vi "attempt-profileStaveCoreHeight.vi"() -> ()   [LabVIEW 2016]
uses:
  <vilib>/vision/driver/NI_Vision_Acquisition_Software.lvlib
  <vilib>/vision/NI_Vision_Development_Module.lvlib
  <vilib>/Utility/file.llb/Read Delimited Spreadsheet (DBL).vi
  <vilib>/Utility/file.llb/Write Delimited Spreadsheet (string).vi
  <vilib>/Utility/file.llb/Write Delimited Spreadsheet (DBL).vi
panel:
  out "True match index vector":i32[](array[numeric])=[1, 1, 1, 1, 1, 1, 1, 1, 1, 1, 1, 1, 1, 1, 1, 1, 1, 1, 1, 1, 1, 1, 1, 1, 1, 1, 1, 1, 1, 1, 1, 1, 1, 1, 1, 1, 1, 1, 1, 1, 1, 1, 1, 1, 1, 1, 1, 1, 1, 1, 1, 1, 1, 1, 1, 1, 1, 1, 1, 1, 1, 1, 1, 1, 1, 1, 1, 1, 1, 1, 1, 1, 1, 1, 1, 1, 1, 1, 1, 1, 1, 1, 1, 1, 1, 1, 1, 1, 1, 1, 1, 1, 1, 1, 1, 1, 1, 1, 1, 1, 1]
  in  "Save plots file path":path=path "E:/XYZstage+Camera_CollectedImages/12-14-2016"
  out "Z displacement [mm]":dbl[](array[numeric])=[-2.0, -1.9, -1.8, -1.7, -1.6, -1.5, -1.4, -1.2999999999999998, -1.2, -1.1, -1.0, -0.8999999999999999, -0.7999999999999998, -0.7, -0.5999999999999999, -0.5, -0.3999999999999999, -0.2999999999999998, -0.19999999999999996, -0.09999999999999987, 0.0, 0.10000000000000009, 0.20000000000000018, 0.30000000000000027, 0.40000000000000036, 0.5, 0.6000000000000001, 0.7000000000000002, 0.8000000000000003, 0.9000000000000004, 1.0, 1.1, 1.2000000000000002, 1.3000000000000003, 1.4000000000000004, 1.5, 1.6, 1.7000000000000002, 1.8000000000000003, 1.9000000000000004, 2.0, 2.1000000000000005, 2.2, 2.3, 2.4000000000000004, 2.5, 2.6000000000000005, 2.7, 2.8000000000000007, 2.9000000000000004, 3.0, 3.1000000000000005, 3.2, 3.3000000000000007, 3.4000000000000004, 3.5, 3.6000000000000005, 3.7, 3.8000000000000007, 3.9000000000000004, 4.0, 4.1000000000000005, 4.2, 4.300000000000001, 4.4, 4.5, 4.6000000000000005, 4.7, 4.800000000000001, 4.9, 5.0, 5.1000000000000005, 5.2, 5.300000000000001, 5.4, 5.5, 5.6000000000000005, 5.7, 5.800000000000001, 5.9, 6.0, 6.1, 6.200000000000001, 6.300000000000001, 6.4, 6.5, 6.6, 6.700000000000001, 6.800000000000001, 6.9, 7.0, 7.1, 7.200000000000001, 7.300000000000001, 7.4, 7.5, 7.600000000000001, 7.700000000000001, 7.800000000000001, 7.9, 8.0]
  out "Line Profile SD vs displacement":cluster{dbl[], sgl[]}(graph)={[-2.0, -1.9, -1.8, -1.7, -1.6, -1.5, -1.4, -1.2999999999999998, -1.2, -1.1, -1.0, -0.8999999999999999, -0.7999999999999998, -0.7, -0.5999999999999999, -0.5, -0.3999999999999999, -0.2999999999999998, -0.19999999999999996, -0.09999999999999987, 0.0, 0.10000000000000009, 0.20000000000000018, 0.30000000000000027, 0.40000000000000036, 0.5, 0.6000000000000001, 0.7000000000000002, 0.8000000000000003, 0.9000000000000004, 1.0, 1.1, 1.2000000000000002, 1.3000000000000003, 1.4000000000000004, 1.5, 1.6, 1.7000000000000002, 1.8000000000000003, 1.9000000000000004, 2.0, 2.1000000000000005, 2.2, 2.3, 2.4000000000000004, 2.5, 2.6000000000000005, 2.7, 2.8000000000000007, 2.9000000000000004, 3.0, 3.1000000000000005, 3.2, 3.3000000000000007, 3.4000000000000004, 3.5, 3.6000000000000005, 3.7, 3.8000000000000007, 3.9000000000000004, 4.0, 4.1000000000000005, 4.2, 4.300000000000001, 4.4, 4.5, 4.6000000000000005, 4.7, 4.800000000000001, 4.9, 5.0, 5.1000000000000005, 5.2, 5.300000000000001, 5.4, 5.5, 5.6000000000000005, 5.7, 5.800000000000001, 5.9, 6.0, 6.1, 6.200000000000001, 6.300000000000001, 6.4, 6.5, 6.6, 6.700000000000001, 6.800000000000001, 6.9, 7.0, 7.1, 7.200000000000001, 7.300000000000001, 7.4, 7.5, 7.600000000000001, 7.700000000000001, 7.800000000000001, 7.9, 8.0], [13.778814, 13.832154, 13.818352, 13.810552, 13.883811, 13.894283, 13.899467, 13.916209, 13.933476, 13.961703, 13.955698, 13.9895115, 13.971683, 14.028705, 14.043394, 14.072498, 14.079607, 14.094322, 14.10442, 14.146118, 14.114918, 14.148811, 14.173441, 14.218914, 14.194622, 14.272478, 14.306726, 14.26945, 14.336761, 14.362134, 14.373682, 14.395194, 14.455633, 14.497305, 14.4799185, 14.594659, 14.592479, 14.642527, 14.660905, 14.72331, 14.78993, 14.833229, 14.888031, 14.981282, 15.005414, 15.038977, 15.041095, 15.103504, 15.177525, 15.183865, 15.1743145, 15.172032, 15.142773, 15.190067, 15.161669, 15.174502, 15.0652895, 15.069694, 14.985318, 14.927153, 14.907353, 14.82682, 14.799372, 14.752344, 14.71759, 14.653623, 14.566762, 14.559869, 14.529179, 14.473595, 14.442641, 14.400999, 14.413042, 14.296873, 14.31068, 14.228256, 14.248779, 14.179554, 14.15682, 14.11064, 14.146657, 14.0807495, 14.068824, 14.026832, 14.009014, 14.026801, 14.005717, 13.982046, 13.993479, 13.971404, 13.941189, 13.940967, 13.946141, 13.935011, 13.897868, 13.873486, 13.894711, 13.855465, 13.869112, 13.84076, 13.822611]}
  in  "Line Profile Coordinates":i32[](array[numeric])=[0, 972, 2592, 972]
  out "Line Profile":cluster{"x0":sgl, "dx":sgl, "Pixels Line":sgl[]}(graph)={"x0"=0.0, "dx"=1.0, "Pixels Line"=[30.0, 30.0, 30.0, 29.0, 31.0, 30.0, 30.0, 30.0, 28.0, 30.0, 31.0, 31.0, 29.0, 31.0, 30.0, 31.0, 30.0, 29.0, 31.0, 32.0, 31.0, 31.0, 32.0, 32.0, 32.0, 32.0, 33.0, 33.0, 30.0, 35.0, 32.0, 32.0, 32.0, 33.0, 32.0, 35.0, 30.0, 34.0, 33.0, 34.0, 34.0, 34.0, 34.0, 34.0, 35.0, 35.0, 32.0, 34.0, 36.0, 36.0, 34.0, 36.0, 34.0, 35.0, 33.0, 38.0, 35.0, 34.0, 36.0, 35.0, 35.0, 37.0, 35.0, 37.0, 36.0, 33.0, 33.0, 37.0, 36.0, 37.0, 35.0, 37.0, 37.0, 36.0, 36.0, 37.0, 35.0, 37.0, 37.0, 33.0, 33.0, 35.0, 33.0, 33.0, 34.0, 34.0, 33.0, 34.0, 32.0, 34.0, 34.0, 34.0, 34.0, 35.0, 34.0, 35.0, 33.0, 34.0, 35.0, 34.0, 33.0, 34.0, 34.0, 33.0, 33.0, 32.0, 33.0, 34.0, 34.0, 31.0, 31.0, 31.0, 32.0, 31.0, 33.0, 32.0, 32.0, 31.0, 30.0, 31.0, 31.0, 33.0, 29.0, 32.0, 30.0, 31.0, 31.0, 32.0, 31.0, 30.0, 30.0, 32.0, 30.0, 31.0, 29.0, 31.0, 30.0, 29.0, 30.0, 30.0, 30.0, 31.0, 31.0, 31.0, 30.0, 32.0, 30.0, 31.0, 31.0, 30.0, 31.0, 31.0, 31.0, 33.0, 29.0, 31.0, 30.0, 31.0, 31.0, 32.0, 31.0, 32.0, 31.0, 30.0, 30.0, 31.0, 33.0, 31.0, 33.0, 33.0, 30.0, 33.0, 30.0, 34.0, 32.0, 33.0, 34.0, 34.0, 32.0, 34.0, 34.0, 34.0, 31.0, 36.0, 35.0, 34.0, 36.0, 31.0, 32.0, 33.0, 32.0, 34.0, 32.0, 33.0, 33.0, 33.0, 35.0, 34.0, 33.0, 33.0, 30.0, 36.0, 33.0, 31.0, 33.0, 32.0, 31.0, 33.0, 32.0, 33.0, 32.0, 33.0, 31.0, 31.0, 33.0, 31.0, 32.0, 32.0, 32.0, 32.0, 32.0, 31.0, 34.0, 33.0, 31.0, 33.0, 33.0, 35.0, 35.0, 34.0, 30.0, 34.0, 32.0, 33.0, 34.0, 34.0, 31.0, 32.0, 32.0, 32.0, 31.0, 32.0, 31.0, 31.0, 32.0, 32.0, 31.0, 33.0, 33.0, 31.0, 31.0, 34.0, 30.0, 35.0, 33.0, 33.0, 29.0, 33.0, 31.0, 32.0, 31.0, 33.0, 32.0, 32.0, 31.0, 32.0, 31.0, 33.0, 30.0, 31.0, 29.0, 30.0, 33.0, 31.0, 31.0, 29.0, 32.0, 32.0, 32.0, 29.0, 31.0, 33.0, 30.0, 32.0, 32.0, 31.0, 32.0, 31.0, 32.0, 31.0, 31.0, 32.0, 31.0, 31.0, 30.0, 32.0, 31.0, 32.0, 34.0, 30.0, 29.0, 33.0, 30.0, 30.0, 30.0, 33.0, 31.0, 31.0, 33.0, 32.0, 30.0, 31.0, 30.0, 32.0, 30.0, 32.0, 32.0, 33.0, 32.0, 34.0, 29.0, 33.0, 29.0, 32.0, 31.0, 32.0, 32.0, 32.0, 33.0, 33.0, 34.0, 32.0, 32.0, 34.0, 33.0, 34.0, 33.0, 34.0, 33.0, 36.0, 33.0, 33.0, 34.0, 34.0, 32.0, 35.0, 32.0, 33.0, 32.0, 32.0, 33.0, 31.0, 33.0, 33.0, 32.0, 36.0, 32.0, 32.0, 32.0, 34.0, 36.0, 32.0, 32.0, 34.0, 33.0, 35.0, 31.0, 32.0, 31.0, 34.0, 37.0, 32.0, 34.0, 35.0, 34.0, 32.0, 33.0, 34.0, 34.0, 34.0, 32.0, 37.0, 32.0, 35.0, 36.0, 35.0, 33.0, 32.0, 31.0, 35.0, 34.0, 34.0, 32.0, 34.0, 34.0, 34.0, 33.0, 33.0, 31.0, 33.0, 33.0, 33.0, 33.0, 34.0, 34.0, 34.0, 33.0, 35.0, 34.0, 34.0, 34.0, 36.0, 32.0, 36.0, 34.0, 35.0, 34.0, 34.0, 33.0, 34.0, 35.0, 37.0, 35.0, 34.0, 35.0, 36.0, 37.0, 36.0, 34.0, 32.0, 35.0, 33.0, 35.0, 35.0, 32.0, 35.0, 34.0, 33.0, 32.0, 33.0, 35.0, 34.0, 34.0, 32.0, 34.0, 33.0, 33.0, 32.0, 32.0, 32.0, 33.0, 33.0, 32.0, 34.0, 33.0, 34.0, 33.0, 34.0, 34.0, 35.0, 32.0, 35.0, 33.0, 33.0, 32.0, 32.0, 34.0, 34.0, 35.0, 34.0, 34.0, 34.0, 36.0, 35.0, 34.0, 35.0, 35.0, 36.0, 36.0, 37.0, 36.0, 35.0, 36.0, 35.0, 35.0, 34.0, 34.0, 35.0, 35.0, 35.0, 36.0, 38.0, 34.0, 34.0, 35.0, 36.0, 34.0, 35.0, 36.0, 35.0, 35.0, 36.0, 34.0, 36.0, 34.0, 36.0, 33.0, 32.0, 36.0, 36.0, 36.0, 35.0, 33.0, 36.0, 33.0, 32.0, 32.0, 35.0, 34.0, 35.0, 33.0, 35.0, 35.0, 34.0, 35.0, 35.0, 37.0, 34.0, 35.0, 35.0, 36.0, 35.0, 34.0, 35.0, 36.0, 35.0, 37.0, 37.0, 36.0, 39.0, 36.0, 37.0, 38.0, 37.0, 37.0, 35.0, 38.0, 40.0, 38.0, 40.0, 36.0, 39.0, 40.0, 37.0, 38.0, 41.0, 37.0, 41.0, 39.0, 41.0, 39.0, 41.0, 39.0, 40.0, 42.0, 40.0, 36.0, 40.0, 40.0, 40.0, 39.0, 40.0, 41.0, 39.0, 38.0, 39.0, 38.0, 39.0, 37.0, 35.0, 35.0, 36.0, 38.0, 36.0, 36.0, 35.0, 36.0, 34.0, 34.0, 35.0, 34.0, 36.0, 33.0, 34.0, 34.0, 32.0, 34.0, 34.0, 33.0, 35.0, 36.0, 35.0, 35.0, 35.0, 35.0, 33.0, 36.0, 33.0, 34.0, 34.0, 34.0, 35.0, 33.0, 35.0, 35.0, 37.0, 36.0, 35.0, 34.0, 33.0, 36.0, 35.0, 34.0, 35.0, 35.0, 34.0, 37.0, 34.0, 37.0, 34.0, 33.0, 35.0, 35.0, 35.0, 36.0, 34.0, 34.0, 35.0, 34.0, 36.0, 34.0, 35.0, 34.0, 35.0, 34.0, 34.0, 38.0, 35.0, 36.0, 37.0, 41.0, 38.0, 37.0, 36.0, 36.0, 39.0, 35.0, 38.0, 37.0, 35.0, 36.0, 36.0, 36.0, 35.0, 33.0, 35.0, 36.0, 32.0, 34.0, 34.0, 34.0, 33.0, 32.0, 30.0, 31.0, 32.0, 30.0, 33.0, 29.0, 31.0, 30.0, 28.0, 28.0, 29.0, 28.0, 28.0, 28.0, 27.0, 28.0, 26.0, 25.0, 24.0, 26.0, 28.0, 26.0, 29.0, 24.0, 25.0, 24.0, 23.0, 23.0, 22.0, 21.0, 20.0, 21.0, 20.0, 18.0, 20.0, 17.0, 19.0, 18.0, 17.0, 17.0, 17.0, 17.0, 15.0, 16.0, 16.0, 14.0, 14.0, 13.0, 12.0, 11.0, 13.0, 12.0, 11.0, 11.0, 11.0, 10.0, 10.0, 10.0, 9.0, 9.0, 9.0, 8.0, 8.0, 8.0, 9.0, 7.0, 7.0, 7.0, 7.0, 7.0, 7.0, 6.0, 6.0, 6.0, 7.0, 7.0, 6.0, 5.0, 6.0, 5.0, 5.0, 5.0, 5.0, 5.0, 5.0, 4.0, 4.0, 4.0, 4.0, 4.0, 4.0, 4.0, 3.0, 4.0, 4.0, 4.0, 3.0, 4.0, 3.0, 3.0, 4.0, 3.0, 3.0, 4.0, 3.0, 4.0, 3.0, 3.0, 3.0, 3.0, 3.0, 3.0, 3.0, 3.0, 3.0, 3.0, 3.0, 3.0, 2.0, 4.0, 3.0, 3.0, 3.0, 3.0, 3.0, 3.0, 3.0, 2.0, 3.0, 3.0, 3.0, 3.0, 2.0, 3.0, 2.0, 3.0, 3.0, 2.0, 3.0, 2.0, 2.0, 3.0, 3.0, 3.0, 3.0, 2.0, 3.0, 2.0, 4.0, 3.0, 3.0, 3.0, 3.0, 4.0, 4.0, 3.0, 3.0, 4.0, 4.0, 3.0, 3.0, 3.0, 4.0, 3.0, 3.0, 3.0, 4.0, 4.0, 3.0, 3.0, 4.0, 3.0, 4.0, 4.0, 3.0, 4.0, 4.0, 4.0, 3.0, 4.0, 4.0, 3.0, 3.0, 3.0, 4.0, 4.0, 4.0, 3.0, 3.0, 3.0, 4.0, 3.0, 3.0, 4.0, 3.0, 3.0, 3.0, 4.0, 3.0, 3.0, 3.0, 3.0, 3.0, 2.0, 3.0, 3.0, 2.0, 4.0, 4.0, 3.0, 3.0, 3.0, 3.0, 3.0, 3.0, 3.0, 3.0, 4.0, 3.0, 3.0, 3.0, 3.0, 3.0, 3.0, 3.0, 2.0, 3.0, 3.0, 3.0, 3.0, 3.0, 3.0, 4.0, 4.0, 3.0, 3.0, 2.0, 4.0, 4.0, 3.0, 3.0, 3.0, 3.0, 2.0, 3.0, 3.0, 3.0, 2.0, 4.0, 3.0, 4.0, 3.0, 3.0, 3.0, 3.0, 3.0, 3.0, 3.0, 3.0, 2.0, 3.0, 3.0, 3.0, 3.0, 4.0, 3.0, 3.0, 3.0, 3.0, 3.0, 4.0, 3.0, 3.0, 3.0, 3.0, 3.0, 4.0, 3.0, 3.0, 3.0, 3.0, 3.0, 3.0, 3.0, 4.0, 3.0, 5.0, 3.0, 5.0, 3.0, 3.0, 3.0, 4.0, 4.0, 4.0, 3.0, 4.0, 5.0, 4.0, 5.0, 6.0, 6.0, 6.0, 7.0, 8.0, 7.0, 7.0, 8.0, 10.0, 9.0, 11.0, 10.0, 13.0, 13.0, 13.0, 13.0, 14.0, 14.0, 16.0, 17.0, 19.0, 17.0, 18.0, 19.0, 19.0, 20.0, 22.0, 22.0, 21.0, 22.0, 21.0, 23.0, 25.0, 25.0, 26.0, 26.0, 29.0, 29.0, 30.0, 29.0, 28.0, 29.0, 32.0, 31.0, 31.0, 31.0, 35.0, 33.0, 35.0, 35.0, 33.0, 34.0, 35.0, 36.0, 35.0, 37.0, 37.0, 38.0, 40.0, 36.0, 40.0, 38.0, 40.0, 39.0, 37.0, 42.0, 41.0, 40.0, 41.0, 39.0, 41.0, 41.0, 42.0, 41.0, 38.0, 42.0, 42.0, 41.0, 40.0, 41.0, 44.0, 38.0, 41.0, 40.0, 43.0, 40.0, 44.0, 42.0, 41.0, 43.0, 43.0, 42.0, 41.0, 44.0, 44.0, 44.0, 45.0, 45.0, 43.0, 46.0, 44.0, 45.0, 42.0, 46.0, 44.0, 44.0, 43.0, 43.0, 46.0, 44.0, 45.0, 44.0, 44.0, 43.0, 44.0, 44.0, 45.0, 45.0, 44.0, 43.0, 43.0, 42.0, 42.0, 44.0, 43.0, 46.0, 43.0, 44.0, 42.0, 42.0, 44.0, 44.0, 43.0, 44.0, 45.0, 44.0, 47.0, 44.0, 46.0, 45.0, 43.0, 44.0, 44.0, 44.0, 43.0, 46.0, 42.0, 43.0, 46.0, 43.0, 47.0, 46.0, 48.0, 44.0, 48.0, 44.0, 43.0, 44.0, 43.0, 44.0, 46.0, 46.0, 45.0, 44.0, 50.0, 46.0, 45.0, 44.0, 45.0, 46.0, 45.0, 41.0, 46.0, 47.0, 47.0, 47.0, 48.0, 46.0, 47.0, 45.0, 44.0, 44.0, 46.0, 43.0, 48.0, 47.0, 45.0, 44.0, 43.0, 44.0, 44.0, 46.0, 46.0, 43.0, 43.0, 43.0, 44.0, 43.0, 44.0, 43.0, 45.0, 46.0, 46.0, 45.0, 45.0, 41.0, 44.0, 42.0, 45.0, 43.0, 47.0, 43.0, 48.0, 46.0, 46.0, 45.0, 46.0, 42.0, 47.0, 43.0, 45.0, 43.0, 45.0, 46.0, 46.0, 45.0, 46.0, 47.0, 47.0, 46.0, 49.0, 48.0, 48.0, 48.0, 50.0, 48.0, 49.0, 52.0, 51.0, 52.0, 52.0, 51.0, 53.0, 52.0, 50.0, 52.0, 50.0, 49.0, 50.0, 49.0, 49.0, 49.0, 54.0, 50.0, 47.0, 49.0, 46.0, 48.0, 48.0, 47.0, 50.0, 51.0, 50.0, 50.0, 49.0, 50.0, 50.0, 47.0, 47.0, 47.0, 44.0, 46.0, 46.0, 45.0, 45.0, 45.0, 47.0, 45.0, 45.0, 43.0, 41.0, 39.0, 37.0, 40.0, 37.0, 36.0, 35.0, 36.0, 37.0, 33.0, 35.0, 31.0, 33.0, 29.0, 27.0, 25.0, 27.0, 25.0, 24.0, 24.0, 24.0, 22.0, 22.0, 20.0, 19.0, 19.0, 18.0, 15.0, 15.0, 15.0, 15.0, 13.0, 12.0, 11.0, 12.0, 8.0, 8.0, 9.0, 8.0, 6.0, 7.0, 6.0, 6.0, 6.0, 5.0, 4.0, 5.0, 5.0, 3.0, 4.0, 5.0, 4.0, 4.0, 3.0, 5.0, 4.0, 3.0, 4.0, 3.0, 4.0, 3.0, 3.0, 3.0, 3.0, 4.0, 3.0, 3.0, 2.0, 4.0, 3.0, 3.0, 2.0, 2.0, 4.0, 3.0, 3.0, 3.0, 4.0, 3.0, 2.0, 3.0, 3.0, 3.0, 3.0, 3.0, 4.0, 3.0, 3.0, 3.0, 3.0, 3.0, 3.0, 3.0, 3.0, 3.0, 3.0, 3.0, 4.0, 3.0, 3.0, 3.0, 3.0, 3.0, 3.0, 3.0, 3.0, 3.0, 3.0, 2.0, 3.0, 3.0, 4.0, 3.0, 3.0, 4.0, 2.0, 3.0, 3.0, 3.0, 3.0, 3.0, 2.0, 3.0, 3.0, 4.0, 3.0, 3.0, 3.0, 3.0, 3.0, 3.0, 3.0, 3.0, 2.0, 3.0, 2.0, 4.0, 2.0, 3.0, 2.0, 3.0, 3.0, 3.0, 3.0, 3.0, 3.0, 3.0, 2.0, 3.0, 2.0, 3.0, 3.0, 3.0, 3.0, 3.0, 4.0, 3.0, 3.0, 3.0, 2.0, 3.0, 3.0, 3.0, 3.0, 3.0, 3.0, 3.0, 2.0, 3.0, 3.0, 3.0, 3.0, 3.0, 3.0, 3.0, 3.0, 3.0, 2.0, 3.0, 3.0, 2.0, 2.0, 3.0, 2.0, 3.0, 2.0, 3.0, 3.0, 2.0, 3.0, 2.0, 3.0, 3.0, 3.0, 3.0, 3.0, 3.0, 3.0, 3.0, 2.0, 3.0, 2.0, 2.0, 3.0, 3.0, 3.0, 3.0, 4.0, 4.0, 2.0, 3.0, 3.0, 3.0, 3.0, 2.0, 2.0, 2.0, 3.0, 2.0, 3.0, 2.0, 2.0, 2.0, 3.0, 3.0, 4.0, 3.0, 3.0, 3.0, 3.0, 3.0, 3.0, 2.0, 3.0, 3.0, 3.0, 3.0, 3.0, 3.0, 3.0, 3.0, 3.0, 3.0, 3.0, 2.0, 3.0, 3.0, 2.0, 3.0, 3.0, 4.0, 3.0, 3.0, 3.0, 3.0, 4.0, 3.0, 3.0, 4.0, 3.0, 3.0, 4.0, 4.0, 4.0, 5.0, 4.0, 5.0, 4.0, 5.0, 5.0, 5.0, 5.0, 6.0, 6.0, 6.0, 6.0, 6.0, 5.0, 7.0, 7.0, 7.0, 9.0, 7.0, 8.0, 9.0, 9.0, 9.0, 9.0, 9.0, 9.0, 9.0, 11.0, 11.0, 11.0, 11.0, 13.0, 13.0, 12.0, 15.0, 15.0, 14.0, 15.0, 16.0, 17.0, 18.0, 18.0, 21.0, 20.0, 20.0, 21.0, 21.0, 21.0, 23.0, 23.0, 23.0, 26.0, 26.0, 26.0, 28.0, 32.0, 30.0, 32.0, 33.0, 35.0, 36.0, 37.0, 35.0, 38.0, 38.0, 41.0, 41.0, 40.0, 43.0, 42.0, 44.0, 42.0, 42.0, 44.0, 42.0, 41.0, 41.0, 40.0, 38.0, 38.0, 40.0, 38.0, 38.0, 39.0, 37.0, 37.0, 38.0, 37.0, 37.0, 36.0, 36.0, 36.0, 36.0, 36.0, 37.0, 34.0, 36.0, 37.0, 38.0, 37.0, 36.0, 36.0, 38.0, 36.0, 36.0, 34.0, 36.0, 37.0, 36.0, 37.0, 36.0, 39.0, 37.0, 38.0, 38.0, 37.0, 40.0, 41.0, 40.0, 37.0, 38.0, 40.0, 40.0, 38.0, 37.0, 42.0, 40.0, 40.0, 39.0, 38.0, 40.0, 41.0, 40.0, 38.0, 40.0, 40.0, 40.0, 41.0, 41.0, 39.0, 39.0, 41.0, 42.0, 40.0, 42.0, 41.0, 40.0, 40.0, 40.0, 40.0, 40.0, 39.0, 41.0, 40.0, 41.0, 38.0, 38.0, 38.0, 40.0, 38.0, 38.0, 40.0, 36.0, 39.0, 39.0, 38.0, 37.0, 36.0, 38.0, 39.0, 39.0, 37.0, 39.0, 37.0, 40.0, 39.0, 38.0, 37.0, 39.0, 38.0, 37.0, 40.0, 40.0, 36.0, 38.0, 39.0, 39.0, 37.0, 39.0, 39.0, 40.0, 40.0, 41.0, 37.0, 40.0, 41.0, 39.0, 38.0, 40.0, 39.0, 39.0, 38.0, 41.0, 40.0, 38.0, 37.0, 38.0, 37.0, 39.0, 38.0, 38.0, 38.0, 37.0, 38.0, 36.0, 37.0, 38.0, 37.0, 36.0, 36.0, 39.0, 37.0, 35.0, 35.0, 37.0, 36.0, 34.0, 32.0, 34.0, 36.0, 34.0, 34.0, 36.0, 37.0, 35.0, 34.0, 36.0, 35.0, 37.0, 37.0, 36.0, 35.0, 34.0, 36.0, 35.0, 33.0, 35.0, 33.0, 35.0, 35.0, 36.0, 32.0, 36.0, 34.0, 34.0, 34.0, 34.0, 35.0, 33.0, 32.0, 33.0, 33.0, 32.0, 32.0, 31.0, 32.0, 32.0, 33.0, 31.0, 33.0, 32.0, 32.0, 32.0, 32.0, 34.0, 32.0, 34.0, 33.0, 33.0, 31.0, 33.0, 33.0, 32.0, 32.0, 31.0, 32.0, 33.0, 32.0, 30.0, 32.0, 31.0, 30.0, 32.0, 30.0, 30.0, 29.0, 29.0, 30.0, 28.0, 29.0, 32.0, 30.0, 29.0, 31.0, 30.0, 30.0, 30.0, 28.0, 29.0, 28.0, 28.0, 28.0, 30.0, 27.0, 27.0, 29.0, 27.0, 30.0, 28.0, 28.0, 30.0, 29.0, 29.0, 28.0, 27.0, 28.0, 28.0, 27.0, 25.0, 28.0, 29.0, 28.0, 27.0, 26.0, 25.0, 27.0, 27.0, 28.0, 26.0, 27.0, 27.0, 27.0, 27.0, 25.0, 28.0, 25.0, 25.0, 24.0, 25.0, 23.0, 26.0, 24.0, 25.0, 25.0, 25.0, 23.0, 26.0, 24.0, 25.0, 25.0, 25.0, 26.0, 25.0, 25.0, 26.0, 24.0, 24.0, 24.0, 24.0, 23.0, 24.0, 24.0, 23.0, 22.0, 24.0, 23.0, 21.0, 23.0, 22.0, 22.0, 21.0, 21.0, 21.0, 19.0, 19.0, 19.0, 19.0, 19.0, 21.0, 18.0, 18.0, 17.0, 19.0, 18.0, 18.0, 17.0, 17.0, 18.0, 17.0, 17.0, 18.0, 18.0, 19.0, 18.0, 17.0, 18.0, 17.0, 18.0, 17.0, 18.0, 18.0, 17.0, 17.0, 18.0, 19.0, 18.0, 18.0, 17.0, 18.0, 17.0, 16.0, 17.0, 17.0, 18.0, 17.0, 16.0, 16.0, 17.0, 17.0, 17.0, 17.0, 17.0, 17.0, 17.0, 16.0, 16.0, 16.0, 17.0, 17.0, 17.0, 17.0, 16.0, 16.0, 16.0, 17.0, 19.0, 17.0, 15.0, 15.0, 16.0, 17.0, 16.0, 17.0, 16.0, 15.0, 15.0, 16.0, 15.0, 15.0, 16.0, 17.0, 17.0, 15.0, 15.0, 16.0, 16.0, 17.0, 16.0, 16.0, 16.0, 17.0, 15.0, 17.0, 15.0, 16.0, 16.0, 15.0, 16.0, 15.0, 15.0, 16.0, 14.0, 15.0, 16.0, 17.0, 16.0, 16.0, 17.0, 16.0, 16.0, 18.0, 17.0, 15.0, 15.0, 15.0, 16.0, 16.0, 13.0, 16.0, 16.0, 16.0, 16.0, 16.0, 15.0, 16.0, 15.0, 16.0, 16.0, 16.0, 15.0, 15.0, 15.0, 17.0, 15.0, 16.0, 17.0, 16.0, 16.0, 17.0, 16.0, 17.0, 14.0, 15.0, 15.0, 16.0, 18.0, 14.0, 15.0, 15.0, 15.0, 17.0, 16.0, 16.0, 16.0, 14.0, 16.0, 15.0, 15.0, 14.0, 17.0, 15.0, 13.0, 15.0, 14.0, 14.0, 14.0, 15.0, 15.0, 15.0, 16.0, 14.0, 15.0, 15.0, 16.0, 15.0, 15.0, 15.0, 14.0, 15.0, 15.0, 14.0, 15.0, 14.0, 15.0, 15.0, 15.0, 16.0, 14.0, 15.0, 15.0, 15.0, 15.0, 15.0, 15.0, 15.0, 15.0, 15.0, 15.0, 14.0, 16.0, 15.0, 14.0, 14.0, 16.0, 14.0, 13.0, 15.0, 15.0, 15.0, 15.0, 15.0, 14.0, 14.0, 14.0, 15.0, 14.0, 15.0, 15.0, 15.0, 15.0, 15.0, 15.0, 15.0, 15.0, 15.0, 14.0, 15.0, 16.0, 16.0, 15.0, 15.0, 15.0, 17.0, 14.0, 16.0, 14.0, 15.0, 15.0, 13.0, 14.0, 16.0, 15.0, 15.0, 14.0, 16.0, 15.0, 15.0, 16.0, 16.0, 15.0, 15.0, 13.0, 16.0, 15.0, 14.0, 14.0, 14.0, 14.0, 15.0, 15.0, 13.0, 15.0, 15.0, 16.0, 14.0, 13.0, 14.0, 15.0, 14.0, 15.0, 15.0, 14.0, 15.0, 13.0, 16.0, 13.0, 15.0, 13.0, 14.0, 14.0, 13.0, 15.0, 15.0, 14.0, 15.0, 15.0, 15.0, 14.0, 15.0, 14.0, 14.0, 14.0, 14.0, 15.0, 14.0, 15.0, 14.0, 14.0, 13.0, 15.0, 14.0, 14.0, 15.0, 13.0, 13.0, 14.0, 14.0, 14.0, 15.0, 13.0, 14.0, 12.0, 13.0, 12.0, 13.0, 13.0, 13.0, 13.0, 11.0, 13.0, 13.0, 13.0, 13.0, 13.0, 12.0, 12.0, 12.0, 14.0, 14.0, 15.0, 13.0, 13.0, 13.0, 13.0, 13.0, 13.0, 14.0, 14.0, 14.0, 13.0, 13.0, 12.0, 13.0, 12.0, 13.0, 14.0, 13.0, 13.0, 13.0, 14.0, 14.0, 12.0, 13.0, 13.0, 14.0, 12.0, 13.0, 14.0, 14.0, 12.0, 15.0, 13.0, 13.0, 12.0, 14.0, 13.0, 13.0, 13.0, 14.0, 13.0, 14.0, 13.0, 14.0, 14.0, 15.0, 13.0, 14.0, 14.0, 14.0, 14.0, 13.0, 13.0, 14.0, 13.0, 13.0, 12.0, 13.0, 14.0, 13.0, 13.0, 13.0, 12.0, 12.0, 13.0, 13.0, 13.0, 13.0, 12.0, 15.0, 11.0, 13.0, 12.0, 12.0, 11.0, 14.0, 12.0, 14.0, 12.0, 14.0, 13.0, 12.0, 12.0, 12.0, 13.0, 12.0, 12.0, 13.0, 12.0, 12.0, 13.0, 13.0, 12.0, 13.0, 13.0, 13.0, 13.0, 13.0, 13.0, 13.0, 13.0, 12.0, 10.0, 14.0, 12.0, 11.0, 11.0, 12.0, 12.0, 13.0, 13.0, 12.0, 12.0, 13.0, 12.0, 12.0, 12.0, 12.0, 11.0, 13.0, 12.0, 12.0, 14.0, 12.0, 13.0, 13.0, 11.0, 12.0, 12.0, 12.0, 12.0, 12.0, 13.0, 12.0, 11.0, 14.0, 13.0, 13.0, 13.0, 12.0, 12.0, 12.0, 12.0, 13.0, 12.0, 13.0, 12.0, 13.0, 13.0, 12.0, 12.0, 13.0, 11.0, 12.0, 13.0, 14.0, 14.0, 11.0, 13.0, 13.0, 11.0, 11.0, 12.0, 13.0, 13.0, 13.0, 13.0, 12.0, 12.0, 12.0, 11.0, 12.0, 12.0, 12.0, 13.0, 14.0, 14.0, 14.0, 13.0, 13.0, 12.0, 13.0, 12.0, 12.0, 13.0, 13.0, 12.0, 14.0, 13.0, 12.0, 12.0, 13.0, 12.0, 14.0, 14.0, 13.0, 13.0, 13.0, 13.0, 13.0, 12.0, 13.0, 13.0, 13.0, 14.0, 13.0, 14.0, 15.0, 12.0, 13.0, 13.0, 14.0, 13.0, 13.0, 12.0, 12.0, 14.0, 12.0, 13.0, 14.0, 14.0, 14.0, 13.0, 13.0, 13.0, 14.0, 13.0, 14.0, 14.0, 15.0, 12.0, 14.0, 14.0, 13.0, 13.0, 13.0, 13.0, 15.0, 15.0, 13.0, 13.0, 15.0, 15.0, 14.0, 14.0, 13.0, 15.0, 15.0, 13.0, 13.0, 15.0, 13.0, 13.0, 15.0, 15.0, 13.0, 14.0, 13.0, 12.0, 14.0, 12.0, 14.0, 14.0, 14.0, 14.0, 13.0, 13.0, 15.0, 13.0, 13.0, 14.0, 15.0, 14.0, 13.0, 13.0, 14.0, 14.0, 14.0, 15.0, 14.0, 13.0, 15.0, 15.0, 14.0, 13.0, 15.0, 15.0, 15.0, 15.0, 14.0, 13.0, 15.0, 14.0, 14.0, 14.0, 14.0, 13.0, 14.0, 15.0, 15.0, 14.0, 13.0, 15.0, 15.0, 14.0, 14.0, 15.0, 15.0, 13.0, 14.0, 14.0, 14.0, 15.0, 15.0, 13.0, 15.0, 13.0, 14.0, 13.0, 14.0, 14.0, 14.0, 15.0, 14.0, 15.0, 15.0, 14.0, 15.0, 14.0, 13.0, 13.0, 14.0, 14.0, 13.0, 12.0, 14.0, 12.0, 14.0, 13.0, 14.0, 14.0, 14.0, 15.0, 14.0, 14.0, 14.0, 15.0, 15.0, 14.0, 14.0, 14.0, 15.0, 14.0, 14.0, 14.0, 15.0, 14.0, 14.0, 15.0, 14.0, 15.0, 15.0, 13.0, 16.0, 14.0, 15.0]}
  out "Coord. Index":i32
  in  "Process list?":bool
  in  "List of Interesting Locations":path=path "E:/XYZstage+Camera_CollectedImages/12-14-2016/nominalPOS_HighVoltageContacts.csv"
  in  "File delimiter":string=","
  out "Set of Coordinates to Process":dbl[][](array[numeric])=[[-709.0, -32.0, -2.0], [-611.0, -32.0, -2.0], [-513.0, -32.0, -2.0], [-415.0, -32.0, -2.0], [-317.0, -32.0, -2.0], [-219.0, -32.0, -2.0], [-121.0, -32.0, -2.0], [-23.0, -32.0, -2.0], [75.0, -32.0, -2.0], [173.0, -32.0, -2.0], [271.0, -32.0, -2.0], [369.0, -32.0, -2.0], [467.0, -32.0, -2.0], [467.0, -132.0, -2.0], [369.0, -132.0, -2.0], [271.0, -132.0, -2.0], [173.0, -132.0, -2.0], [75.0, -132.0, -2.0], [-23.0, -132.0, -2.0], [-121.0, -132.0, -2.0], [-219.0, -132.0, -2.0], [-317.0, -132.0, -2.0], [-415.0, -132.0, -2.0], [-513.0, -132.0, -2.0], [-611.0, -132.0, -2.0], [-709.0, -132.0, -2.0]]
  out "True match index vs displacement":cluster{dbl[], i32[]}(graph)={[-2.0, -1.9, -1.8, -1.7, -1.6, -1.5, -1.4, -1.2999999999999998, -1.2, -1.1, -1.0, -0.8999999999999999, -0.7999999999999998, -0.7, -0.5999999999999999, -0.5, -0.3999999999999999, -0.2999999999999998, -0.19999999999999996, -0.09999999999999987, 0.0, 0.10000000000000009, 0.20000000000000018, 0.30000000000000027, 0.40000000000000036, 0.5, 0.6000000000000001, 0.7000000000000002, 0.8000000000000003, 0.9000000000000004, 1.0, 1.1, 1.2000000000000002, 1.3000000000000003, 1.4000000000000004, 1.5, 1.6, 1.7000000000000002, 1.8000000000000003, 1.9000000000000004, 2.0, 2.1000000000000005, 2.2, 2.3, 2.4000000000000004, 2.5, 2.6000000000000005, 2.7, 2.8000000000000007, 2.9000000000000004, 3.0, 3.1000000000000005, 3.2, 3.3000000000000007, 3.4000000000000004, 3.5, 3.6000000000000005, 3.7, 3.8000000000000007, 3.9000000000000004, 4.0, 4.1000000000000005, 4.2, 4.300000000000001, 4.4, 4.5, 4.6000000000000005, 4.7, 4.800000000000001, 4.9, 5.0, 5.1000000000000005, 5.2, 5.300000000000001, 5.4, 5.5, 5.6000000000000005, 5.7, 5.800000000000001, 5.9, 6.0, 6.1, 6.200000000000001, 6.300000000000001, 6.4, 6.5, 6.6, 6.700000000000001, 6.800000000000001, 6.9, 7.0, 7.1, 7.200000000000001, 7.300000000000001, 7.4, 7.5, 7.600000000000001, 7.700000000000001, 7.800000000000001, 7.9, 8.0], [1, 1, 1, 1, 1, 1, 1, 1, 1, 1, 1, 1, 1, 1, 1, 1, 1, 1, 1, 1, 1, 1, 1, 1, 1, 1, 1, 1, 1, 1, 1, 1, 1, 1, 1, 1, 1, 1, 1, 1, 1, 1, 1, 1, 1, 1, 1, 1, 1, 1, 1, 1, 1, 1, 1, 1, 1, 1, 1, 1, 1, 1, 1, 1, 1, 1, 1, 1, 1, 1, 1, 1, 1, 1, 1, 1, 1, 1, 1, 1, 1, 1, 1, 1, 1, 1, 1, 1, 1, 1, 1, 1, 1, 1, 1, 1, 1, 1, 1, 1, 1]}
  in  "True position y":sgl=919.0
  in  "True position x":sgl=1107.0
  out "SD Intensity":cluster{dbl[], sgl[]}(graph)={[-2.0, -1.9, -1.8, -1.7, -1.6, -1.5, -1.4, -1.2999999999999998, -1.2, -1.1, -1.0, -0.8999999999999999, -0.7999999999999998, -0.7, -0.5999999999999999, -0.5, -0.3999999999999999, -0.2999999999999998, -0.19999999999999996, -0.09999999999999987, 0.0, 0.10000000000000009, 0.20000000000000018, 0.30000000000000027, 0.40000000000000036, 0.5, 0.6000000000000001, 0.7000000000000002, 0.8000000000000003, 0.9000000000000004, 1.0, 1.1, 1.2000000000000002, 1.3000000000000003, 1.4000000000000004, 1.5, 1.6, 1.7000000000000002, 1.8000000000000003, 1.9000000000000004, 2.0, 2.1000000000000005, 2.2, 2.3, 2.4000000000000004, 2.5, 2.6000000000000005, 2.7, 2.8000000000000007, 2.9000000000000004, 3.0, 3.1000000000000005, 3.2, 3.3000000000000007, 3.4000000000000004, 3.5, 3.6000000000000005, 3.7, 3.8000000000000007, 3.9000000000000004, 4.0, 4.1000000000000005, 4.2, 4.300000000000001, 4.4, 4.5, 4.6000000000000005, 4.7, 4.800000000000001, 4.9, 5.0, 5.1000000000000005, 5.2, 5.300000000000001, 5.4, 5.5, 5.6000000000000005, 5.7, 5.800000000000001, 5.9, 6.0, 6.1, 6.200000000000001, 6.300000000000001, 6.4, 6.5, 6.6, 6.700000000000001, 6.800000000000001, 6.9, 7.0, 7.1, 7.200000000000001, 7.300000000000001, 7.4, 7.5, 7.600000000000001, 7.700000000000001, 7.800000000000001, 7.9, 8.0], [10.641642, 10.651783, 10.666476, 10.678297, 10.692045, 10.704219, 10.71487, 10.729536, 10.741039, 10.750571, 10.763839, 10.775967, 10.788582, 10.799376, 10.81211, 10.824463, 10.83405, 10.845817, 10.859667, 10.870168, 10.882172, 10.89403, 10.906297, 10.919101, 10.931665, 10.943659, 10.956027, 10.969385, 10.981974, 10.995705, 11.010284, 11.024967, 11.0413475, 11.057471, 11.074867, 11.091722, 11.112195, 11.129671, 11.15188, 11.172808, 11.193802, 11.216489, 11.236443, 11.253368, 11.273286, 11.291981, 11.304524, 11.317779, 11.327574, 11.333745, 11.336129, 11.336787, 11.332882, 11.329793, 11.322591, 11.313084, 11.304098, 11.292609, 11.283385, 11.271473, 11.260806, 11.251673, 11.241544, 11.231288, 11.225223, 11.217907, 11.210427, 11.205402, 11.200951, 11.193987, 11.189045, 11.183764, 11.177903, 11.175188, 11.171228, 11.166864, 11.165156, 11.162128, 11.160154, 11.158059, 11.1588125, 11.157321, 11.157779, 11.158607, 11.159854, 11.16267, 11.164532, 11.167459, 11.167222, 11.171898, 11.173964, 11.176909, 11.17766, 11.180899, 11.182198, 11.1821165, 11.183969, 11.183027, 11.185584, 11.186689, 11.18563]}
  out "Mean intensity":cluster{dbl[], sgl[]}(graph)={[-2.0, -1.9, -1.8, -1.7, -1.6, -1.5, -1.4, -1.2999999999999998, -1.2, -1.1, -1.0, -0.8999999999999999, -0.7999999999999998, -0.7, -0.5999999999999999, -0.5, -0.3999999999999999, -0.2999999999999998, -0.19999999999999996, -0.09999999999999987, 0.0, 0.10000000000000009, 0.20000000000000018, 0.30000000000000027, 0.40000000000000036, 0.5, 0.6000000000000001, 0.7000000000000002, 0.8000000000000003, 0.9000000000000004, 1.0, 1.1, 1.2000000000000002, 1.3000000000000003, 1.4000000000000004, 1.5, 1.6, 1.7000000000000002, 1.8000000000000003, 1.9000000000000004, 2.0, 2.1000000000000005, 2.2, 2.3, 2.4000000000000004, 2.5, 2.6000000000000005, 2.7, 2.8000000000000007, 2.9000000000000004, 3.0, 3.1000000000000005, 3.2, 3.3000000000000007, 3.4000000000000004, 3.5, 3.6000000000000005, 3.7, 3.8000000000000007, 3.9000000000000004, 4.0, 4.1000000000000005, 4.2, 4.300000000000001, 4.4, 4.5, 4.6000000000000005, 4.7, 4.800000000000001, 4.9, 5.0, 5.1000000000000005, 5.2, 5.300000000000001, 5.4, 5.5, 5.6000000000000005, 5.7, 5.800000000000001, 5.9, 6.0, 6.1, 6.200000000000001, 6.300000000000001, 6.4, 6.5, 6.6, 6.700000000000001, 6.800000000000001, 6.9, 7.0, 7.1, 7.200000000000001, 7.300000000000001, 7.4, 7.5, 7.600000000000001, 7.700000000000001, 7.800000000000001, 7.9, 8.0], [20.910046, 20.920034, 20.933973, 20.943743, 20.955025, 20.964808, 20.9742, 20.98869, 20.994587, 21.002455, 21.015623, 21.023836, 21.03432, 21.04218, 21.053076, 21.061861, 21.071775, 21.081497, 21.091366, 21.098965, 21.109715, 21.117125, 21.126795, 21.136934, 21.146261, 21.154997, 21.164537, 21.172298, 21.18154, 21.189453, 21.19927, 21.211632, 21.220724, 21.229343, 21.23793, 21.247366, 21.258081, 21.265568, 21.273588, 21.283756, 21.294106, 21.302652, 21.31348, 21.320198, 21.327011, 21.338882, 21.345778, 21.358772, 21.366032, 21.376537, 21.384182, 21.392761, 21.40514, 21.417728, 21.425573, 21.433475, 21.441751, 21.451128, 21.459505, 21.468637, 21.47673, 21.483612, 21.492018, 21.49752, 21.503105, 21.509392, 21.514872, 21.523632, 21.529394, 21.531126, 21.542875, 21.543736, 21.54888, 21.55595, 21.561668, 21.567684, 21.575727, 21.58373, 21.591654, 21.598585, 21.611357, 21.617191, 21.631332, 21.643969, 21.65866, 21.672548, 21.685982, 21.70223, 21.714117, 21.73156, 21.747263, 21.763897, 21.775932, 21.792603, 21.805487, 21.818777, 21.831142, 21.844866, 21.861055, 21.877483, 21.887157]}
  out "Match score vs displacement":cluster{dbl[], sgl[]}(graph)={[-2.0, -1.9, -1.8, -1.7, -1.6, -1.5, -1.4, -1.2999999999999998, -1.2, -1.1, -1.0, -0.8999999999999999, -0.7999999999999998, -0.7, -0.5999999999999999, -0.5, -0.3999999999999999, -0.2999999999999998, -0.19999999999999996, -0.09999999999999987, 0.0, 0.10000000000000009, 0.20000000000000018, 0.30000000000000027, 0.40000000000000036, 0.5, 0.6000000000000001, 0.7000000000000002, 0.8000000000000003, 0.9000000000000004, 1.0, 1.1, 1.2000000000000002, 1.3000000000000003, 1.4000000000000004, 1.5, 1.6, 1.7000000000000002, 1.8000000000000003, 1.9000000000000004, 2.0, 2.1000000000000005, 2.2, 2.3, 2.4000000000000004, 2.5, 2.6000000000000005, 2.7, 2.8000000000000007, 2.9000000000000004, 3.0, 3.1000000000000005, 3.2, 3.3000000000000007, 3.4000000000000004, 3.5, 3.6000000000000005, 3.7, 3.8000000000000007, 3.9000000000000004, 4.0, 4.1000000000000005, 4.2, 4.300000000000001, 4.4, 4.5, 4.6000000000000005, 4.7, 4.800000000000001, 4.9, 5.0, 5.1000000000000005, 5.2, 5.300000000000001, 5.4, 5.5, 5.6000000000000005, 5.7, 5.800000000000001, 5.9, 6.0, 6.1, 6.200000000000001, 6.300000000000001, 6.4, 6.5, 6.6, 6.700000000000001, 6.800000000000001, 6.9, 7.0, 7.1, 7.200000000000001, 7.300000000000001, 7.4, 7.5, 7.600000000000001, 7.700000000000001, 7.800000000000001, 7.9, 8.0], [879.0314, 880.5322, 881.50525, 883.59375, 885.04114, 886.6321, 887.99164, 889.89014, 891.54895, 892.7096, 894.01355, 895.76086, 896.38574, 897.8513, 899.14215, 900.46564, 901.9159, 903.5967, 905.61066, 907.6271, 909.8519, 911.7539, 914.30066, 916.9432, 919.2109, 922.02893, 925.1449, 927.1994, 930.3543, 933.7616, 937.412, 941.27527, 945.56866, 949.7169, 954.40594, 958.87146, 964.12915, 966.3607, 971.17303, 975.7742, 979.7761, 983.59674, 986.48694, 988.4218, 989.78876, 991.7045, 990.82227, 992.4532, 993.7908, 994.56085, 994.9838, 995.4237, 995.7052, 996.1429, 996.40594, 995.1158, 994.9518, 994.49426, 993.5686, 991.30493, 988.9285, 985.62024, 979.23346, 976.25146, 972.1395, 967.325, 962.50824, 957.11816, 951.9495, 947.2621, 943.3269, 939.42737, 936.4822, 934.05096, 931.73193, 929.0479, 926.9251, 923.81866, 921.44275, 919.72864, 917.4266, 914.7757, 913.0611, 911.3056, 910.391, 910.2793, 909.92053, 909.1891, 908.61414, 907.92114, 906.2847, 905.24835, 904.1167, 902.81866, 901.4715, 900.2599, 898.7702, 897.3308, 896.09454, 894.80115, 893.3429]}
  in  "Match position variation tolerance":sgl=0.25
  out "Z step":dbl=10.0
  out "Image":T1(plugin-control)
  in  "End Z [mm]":dbl=8.0
  in  "Stepsize [mm]":dbl=0.1
  out "Matches (pixel)":T2(array[cluster])=[{"Position"={"x"=1127.198, "y"=915.98065}, "Angle"=0.0, "Scale"=1.0, "Score"=893.3429, "Bounding Box"=[{"x"=974.198, "y"=763.98065}, {"x"=1280.198, "y"=763.98065}, {"x"=1280.198, "y"=1067.9807}, {"x"=974.198, "y"=1067.9807}, {"x"=974.198, "y"=763.98065}]}, {"Position"={"x"=1514.1495, "y"=359.13376}, "Angle"=0.0, "Scale"=1.0, "Score"=588.01715, "Bounding Box"=[{"x"=1361.1495, "y"=207.13376}, {"x"=1667.1495, "y"=207.13376}, {"x"=1667.1495, "y"=511.13376}, {"x"=1361.1495, "y"=511.13376}, {"x"=1361.1495, "y"=207.13376}]}, {"Position"={"x"=530.31506, "y"=1381.0135}, "Angle"=0.0, "Scale"=1.0, "Score"=572.6888, "Bounding Box"=[{"x"=377.31506, "y"=1229.0135}, {"x"=683.31506, "y"=1229.0135}, {"x"=683.31506, "y"=1533.0135}, {"x"=377.31506, "y"=1533.0135}, {"x"=377.31506, "y"=1229.0135}]}, {"Position"={"x"=1194.1893, "y"=1528.8197}, "Angle"=0.0, "Scale"=1.0, "Score"=556.0711, "Bounding Box"=[{"x"=1041.1893, "y"=1376.8197}, {"x"=1347.1893, "y"=1376.8197}, {"x"=1347.1893, "y"=1680.8197}, {"x"=1041.1893, "y"=1680.8197}, {"x"=1041.1893, "y"=1376.8197}]}, {"Position"={"x"=129.51509, "y"=1364.8577}, "Angle"=0.0, "Scale"=1.0, "Score"=534.0569, "Bounding Box"=[{"x"=-23.48491, "y"=1212.8577}, {"x"=282.51508, "y"=1212.8577}, {"x"=282.51508, "y"=1516.8577}, {"x"=-23.48491, "y"=1516.8577}, {"x"=-23.48491, "y"=1212.8577}]}, {"Position"={"x"=1668.3909, "y"=1350.8374}, "Angle"=0.0, "Scale"=1.0, "Score"=523.21924, "Bounding Box"=[{"x"=1515.3909, "y"=1198.8374}, {"x"=1821.3909, "y"=1198.8374}, {"x"=1821.3909, "y"=1502.8374}, {"x"=1515.3909, "y"=1502.8374}, {"x"=1515.3909, "y"=1198.8374}]}, {"Position"={"x"=120.40187, "y"=1854.9404}, "Angle"=0.0, "Scale"=1.0, "Score"=515.30743, "Bounding Box"=[{"x"=-32.59813, "y"=1702.9404}, {"x"=273.40186, "y"=1702.9404}, {"x"=273.40186, "y"=2006.9404}, {"x"=-32.59813, "y"=2006.9404}, {"x"=-32.59813, "y"=1702.9404}]}, {"Position"={"x"=840.2334, "y"=1425.0645}, "Angle"=0.0, "Scale"=1.0, "Score"=508.74185, "Bounding Box"=[{"x"=687.2334, "y"=1273.0645}, {"x"=993.2334, "y"=1273.0645}, {"x"=993.2334, "y"=1577.0645}, {"x"=687.2334, "y"=1577.0645}, {"x"=687.2334, "y"=1273.0645}]}, {"Position"={"x"=1681.2684, "y"=805.9706}, "Angle"=0.0, "Scale"=1.0, "Score"=501.45316, "Bounding Box"=[{"x"=1528.2684, "y"=653.9706}, {"x"=1834.2684, "y"=653.9706}, {"x"=1834.2684, "y"=957.9706}, {"x"=1528.2684, "y"=957.9706}, {"x"=1528.2684, "y"=653.9706}]}] {"Bounding Box"."y" format="%.2f"; "Bounding Box"."x" format="%.2f"; "Score" format="%.2f"; "Scale" format="%.2f"; "Angle" format="%.2f"; "Position"."y" format="%.2f"; "Position"."x" format="%.2f"}
  in  "Match parameters":T3={"Number of Matches Requested"=10, "Minimum Match Score"=500.0, "Angle Ranges"=[]}
  in  "Template File Path":path=path "E:/XYZstage+Camera_CollectedImages/12-14-2016/test_sub_smallerDot_-685,-128,3p4.png"
  in  "Axes Speeds [mm/s]":T4={"X Speed"=25.0, "Y Speed"=5.0, "Z Speed"=1.0}
  in  "Initial Location [mm]":T5={"Go to X"=-685.0, "Go to Y"=-128.0, "Go to Z"=-2.0}
  out "Intensity histogram":T6(graph)={"Starting Value"=0.0, "Incremental Value"=1.0, "Histogram"=[0, 150, 32506, 224440, 72176, 32514, 24980, 20375, 14194, 28017, 104301, 253038, 323157, 301095, 227717, 209323, 173693, 175646, 161707, 128964, 105278, 82020, 84233, 81813, 93253, 96135, 110312, 107820, 127805, 130789, 152441, 156182, 178245, 162226, 149895, 115876, 98993, 74348, 64510, 51354, 47133, 38158, 37497, 33782, 33023, 26163, 21842, 15148, 11810, 8588, 7813, 6201, 4673, 4086, 3220, 2494, 1799, 1446, 1003, 718, 376, 228, 88, 29, 7, 2, 0, 0, 0, 0, 0, 0, 0, 0, 0, 0, 0, 0, 0, 0, 0, 0, 0, 0, 0, 0, 0, 0, 0, 0, 0, 0, 0, 0, 0, 0, 0, 0, 0, 0, 0, 0, 0, 0, 0, 0, 0, 0, 0, 0, 0, 0, 0, 0, 0, 0, 0, 0, 0, 0, 0, 0, 0, 0, 0, 0, 0, 0, 0, 0, 0, 0, 0, 0, 0, 0, 0, 0, 0, 0, 0, 0, 0, 0, 0, 0, 0, 0, 0, 0, 0, 0, 0, 0, 0, 0, 0, 0, 0, 0, 0, 0, 0, 0, 0, 0, 0, 0, 0, 0, 0, 0, 0, 0, 0, 0, 0, 0, 0, 0, 0, 0, 0, 0, 0, 0, 0, 0, 0, 0, 0, 0, 0, 0, 0, 0, 0, 0, 0, 0, 0, 0, 0, 0, 0, 0, 0, 0, 0, 0, 0, 0, 0, 0, 0, 0, 0, 0, 0, 0, 0, 0, 0, 0, 0, 0, 0, 0, 0, 0, 0, 0, 0, 0, 0, 0, 0, 0, 0, 0, 0, 0, 0, 0, 0, 0, 0, 0, 0, 0, 0, 0, 0, 0, 0, 0]}
  out "Moving":bool
  out "XYZ Stage Current Position":T7={"X [-750, 750 mm]"=-684.9998825073242, "Y [-150, 30 mm]"=-128.00212852478026, "Z [-50, 50 mm]"=7.9998000000000005}
  out "Error report":errorcluster
  in  "Camera Name":refnum<k21>="cam0" caption="IMAQdx Session"
  # "ANALYSIS"
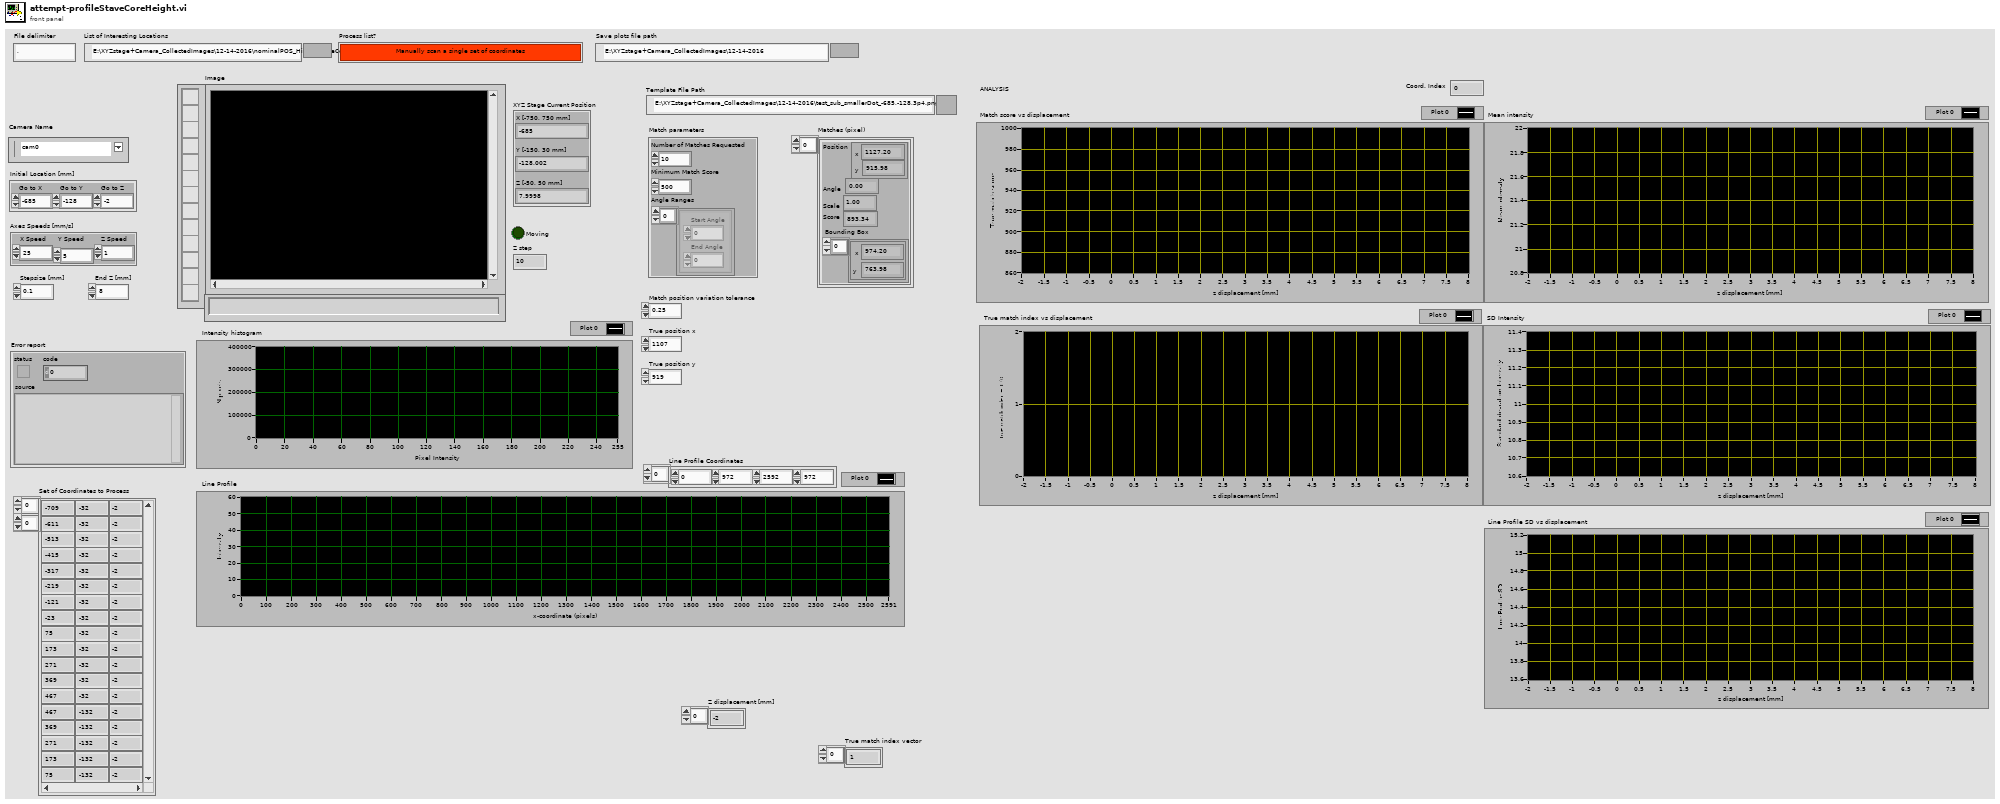
[diagram p1: front panel]
types:
  T1 = typedef "IMAQ Image.ctl" = refnum<image>
  T2 = cluster{"Position":cluster{"x":sgl, "y":sgl}, "Angle":sgl, "Scale":sgl, "Score":sgl, "Bounding Box":cluster{"x":sgl, "y":sgl}[]}[]
  T3 = cluster{"Number of Matches Requested":i32, "Minimum Match Score":sgl, "Angle Ranges":cluster{"Start Angle":sgl, "End Angle":sgl}[]}
  T4 = cluster{"X Speed":dbl, "Y Speed":dbl, "Z Speed":dbl}
  T5 = cluster{"Go to X":dbl, "Go to Y":dbl, "Go to Z":dbl}
  T6 = cluster{"Starting Value":sgl, "Incremental Value":sgl, "Histogram":u32[]}
  T7 = cluster{"X [-750, 750 mm]":dbl, "Y [-150, 30 mm]":dbl, "Z [-50, 50 mm]":dbl}
  T8 = cluster{"Set of Coordinates to Process[0]":dbl, "Set of Coordinates to Process[1]":dbl, "Set of Coordinates to Process[2]":dbl}
  T9 = typedef "Image Type" = u32
  T10 = typedef "IMAQdx.ctl" = refnum<k21>
  T11 = cluster{"Final X":dbl, "Final Y":dbl, "Final Z":dbl}
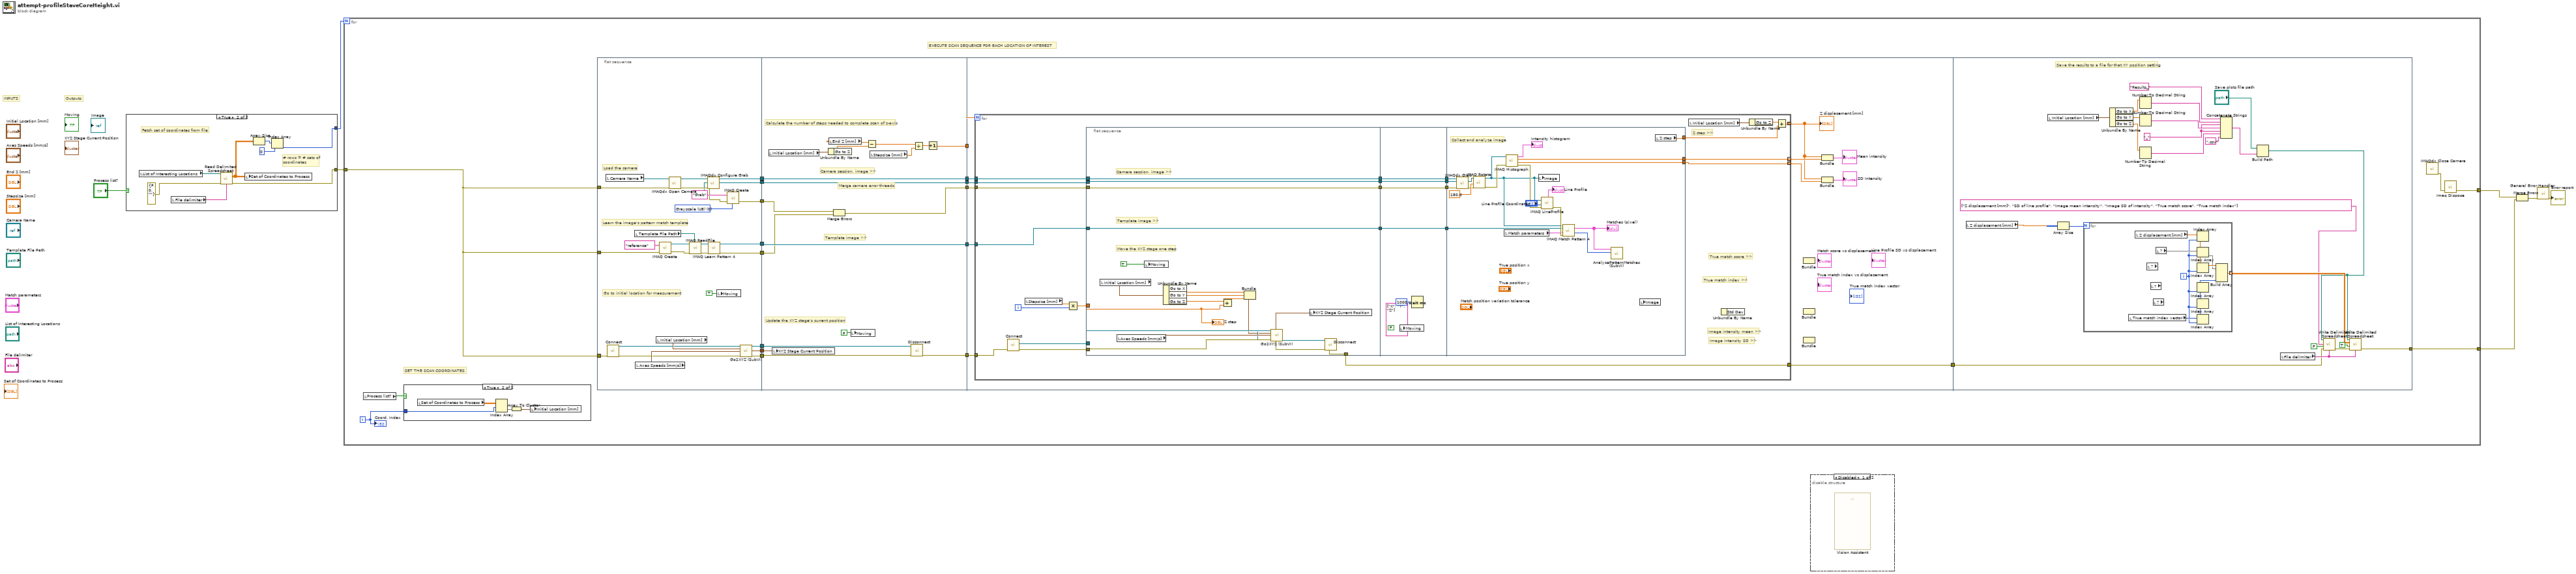
[diagram p0: block diagram]
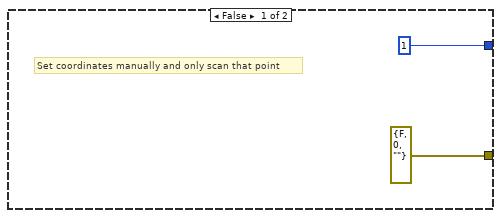
[diagram p2: hidden frame]
diagram:
  # "Outputs"
  # "INPUTS"
  n1 = case shown="True" "Process list?" {
    tunnel: [1 w12] -> w2
    tunnel: [errorcluster {"status"=FALSE, "code"=0, "source"=""} ("error in (no error)") w10] -> w3
    frame False {
      # "Set coordinates manually and only scan that point"
    }
    frame True {
      # "# rows = # sets of\ncoordinates"
      # "Fetch set of coordinates from file"
      n2 = local read "List of Interesting Locations"() -> (w16:path)
      n3 = local read "File delimiter"() -> (w17:string)
      n4 = call-poly <vilib>:"Read Delimited Spreadsheet.vi"("file path (dialog if empty)"=w16, "error in (no error)"=errorcluster {"status"=FALSE, "code"=0, "source"=""}, "delimiter (\\t)"=w17) -> ("all rows"=w15:dbl[][], "error out"=w10:errorcluster)  [unwired: 7 in, 4 out]
      n5 = local write "Set of Coordinates to Process"(w15) -> ()
      n6 = Array Size(array=w15) -> (size(s)=w14:i32[])
      n7 = Index Array(array=w14, index=0) -> (element=w12:i32)
    }
  }
  n8 = for {
    N: w2 -> [_]
    tunnel: [w24] -> w6
    tunnel: w3 -> [w18]
    tunnel: [w19] -> w1
    i -> [w22]
    # "SET THE SCAN COORDINATES"
    # "EXECUTE SCAN SEQUENCE FOR EACH LOCATION OF INTEREST"
    n9 = local read "Process list?"() -> (w23:bool)
    n10 = case shown="True" w23 {
      tunnel: w22 -> [_ w41]
      frame False {
      }
      frame True {
        n11 = local read "Set of Coordinates to Process"() -> (w42:dbl[][])
        n12 = Index Array(array=w42, index (row)=w41) -> (element=w40:dbl[])  [unwired: 1 in]
        n13 = Array To Cluster(array=w40) -> (cluster=w39:T8)
        n14 = local write "Initial Location [mm]"(w39) -> ()
      }
    }
    n15 = flat-sequence {
      tunnel: [w70] -> w38
      tunnel: [w69] -> w37
      tunnel: [w64] -> w36
      tunnel: [w53] -> w35
      tunnel: [w49] -> w34
      tunnel: [w48] -> w33
      tunnel: [w47] -> w32
      tunnel: [w46] -> w31
      tunnel: w18 -> [w45]
      tunnel: w18 -> [w44]
      tunnel: w18 -> [w43]
      tunnel: w38 -> [w83]
      tunnel: w37 -> [w82]
      tunnel: w36 -> [w87]
      tunnel: [w73] -> w30
      tunnel: [w81] -> w29
      tunnel: [w79] -> w28
      tunnel: w35 -> [w79]
      tunnel: w34 -> [w78]
      tunnel: [w78] -> w27
      tunnel: w33 -> [w76]
      tunnel: [w72] -> w26
      tunnel: [w77] -> w25
      tunnel: w32 -> [w77]
      tunnel: w31 -> [w71]
      tunnel: w30 -> [w94]
      tunnel: w29 -> [w100]
      tunnel: w28 -> [w99]
      tunnel: w27 -> [w98]
      tunnel: w26 -> [w97]
      tunnel: w25 -> [w96]
      tunnel: [w95] -> w21
      tunnel: w21 -> [w172]
      tunnel: [w171] -> w19
      frame #0 {
        w51 = T9 0 items=["Grayscale (U8)", "Grayscale (I16)", "Grayscale (SGL)", "Complex (CSG)", "RGB (U32)", "HSL (U32)", "RGB (U64)", "Grayscale (U16)"] ("Image Type")
        # "Learn the image's pattern match template"
        # "Load the camera"
        # "Go to initial location for measurement"
        n16 = local read "Camera Name"() -> (w62:refnum<k21>)
        n17 = call "Connect.vi"("error in (no error)"=w43) -> ("error out"=w63:errorcluster, "controller"=w65:refnum<k24>)  [unwired: 9 in]
        n18 = local read "Template File Path"() -> (w59:path)
        n19 = local read "Axes Speeds [mm/s]"() -> (w67:T4)
        n20 = local read "Initial Location [mm]"() -> (w66:T5)
        n21 = call "IMAQ Create"("Image Name"="reference", "error in (no error)"=w45) -> ("New Image"=w58:T1, "error out"=w57:errorcluster)  [unwired: 3 in]
        n22 = call <vilib>:"IMAQdx Open Camera.vi"("error in"=w44, "Session In"=w62) -> ("error out"=w60:errorcluster, "Session Out"=w61:T10)  [unwired: 1 in, 7 out]
        n23 = call "IMAQ ReadFile"("File Path"=w59, "error in (no error)"=w57, "Image"=w58) -> ("error out"=w54:errorcluster, "Image Out"=w55:T1)  [unwired: 4 in, 3 out]
        n24 = call <vilib>:"IMAQdx Configure Grab.vi"("error in"=w60, "Session In"=w61) -> ("error out"=w50:errorcluster, "Session Out"=w53:T10)  [unwired: 8 out]
        n25 = call "IMAQ Learn Pattern 4"("error in (no error)"=w54, "Image"=w55) -> ("error out"=w46:errorcluster, "Template Image Out"=w47:T1)  [unwired: 7 in, 1 out]
        n26 = local write "Moving"(TRUE ("Moving")) -> ()
        n27 = call "IMAQ Create"("Image Name"="Grab", "Image Type"=w51, "error in (no error)"=w50) -> ("New Image"=w49:T1, "error out"=w48:errorcluster)  [unwired: 1 in, 1 out]
        n28 = call "Go2XYZ (SubVI).vi"(".NET Refnum in"=w65, "Go to Coordinates"=w66, "Axis Speeds"=w67, "error in (no error)"=w63) -> (".NET Refnum out"=w70:refnum<k24>, "Final Position"=w64:T11, "error out"=w69:errorcluster)  [unwired: 8 in, 1 out]
      }
      frame #1 {
        # "Merge camera error threads"
        # "Camera session, image >>"
        # "Template image >>"
        # "Calculate the number of steps needed to complete scan of z-axis"
        # "Update the XYZ stage's current position"
        n29 = local read "Initial Location [mm]"() -> (w86:T5)
        n30 = local write "XYZ Stage Current Position"(w87) -> ()
        n31 = Unbundle By Name(w86) -> ("Go to Z"=w85:dbl)
        n32 = local read "End Z [mm]"() -> (w75:dbl)
        n33 = Merge Errors(w76, w71) -> (w72:errorcluster)
        n34 = local write "Moving"(FALSE ("Moving")) -> ()
        n35 = Subtract(x=w75, y=w85) -> (x-y=w84:dbl)
        n36 = local read "Stepsize [mm]"() -> (w80:dbl)
        n37 = call "Disconnect.vi"("error in (no error)"=w82, "controller"=w83) -> ("error out"=w81:errorcluster)  [unwired: 9 in]
        n38 = Divide(x=w84, y=w80) -> (x/y=w74:dbl)
        n39 = Increment(x=w74) -> (x+1=w73:dbl)
      }
      frame #2 {
        n40 = for {
          N: w94 -> [_]
          tunnel: w100 -> [w122]
          tunnel: w99 -> [w120]
          tunnel: w98 -> [w119]
          tunnel: w97 -> [w118]
          tunnel: w96 -> [w117]
          tunnel: [w116] -> w95
          tunnel: [w114] -> w91 mode=indexing
          tunnel: [w102] -> w93 mode=indexing
          tunnel: [w101] -> w90 mode=indexing
          i -> [w124]
          (unwired) string[] ["X", "Y", "Z"] ("Axes Names")
          # "True match index >>"
          # "Image intensity SD >>"
          # "Image intensity mean >>"
          # "True match score >>"
          # "Z step >>"
          n41 = call "Connect.vi"("error in (no error)"=w122) -> ("error out"=w104:errorcluster, "controller"=w125:refnum<k24>)  [unwired: 9 in]
          n42 = local read "Stepsize [mm]"() -> (w121:dbl)
          n43 = Multiply(x=w121, y=w124) -> (x*y=w123:dbl)
          n44 = flat-sequence {
            tunnel: w125 -> [w144]
            tunnel: w104 -> [w143]
            tunnel: w123 -> [w130]
            tunnel: [w136] -> w112
            tunnel: w120 -> [w136]
            tunnel: w119 -> [w135]
            tunnel: [w135] -> w110
            tunnel: w118 -> [w134]
            tunnel: [w134] -> w108
            tunnel: [w133] -> w106
            tunnel: w117 -> [w133]
            tunnel: [w132] -> w116
            tunnel: w112 -> [w150]
            tunnel: [w150] -> w111
            tunnel: w110 -> [w149]
            tunnel: [w149] -> w109
            tunnel: w108 -> [w148]
            tunnel: [w148] -> w107
            tunnel: w106 -> [w147]
            tunnel: [w147] -> w105
            tunnel: w111 -> [w167]
            tunnel: w109 -> [w168]
            tunnel: w107 -> [w166]
            tunnel: w105 -> [w156]
            tunnel: [w170] -> w103
            tunnel: [w154] -> w102
            tunnel: [w153] -> w101
            frame #0 {
              # "Camera session, image >>"
              # "Template image >>"
              # "Move the XYZ stage one step"
              n45 = local read "Initial Location [mm]"() -> (w140:T5)
              n46 = local read "Axes Speeds [mm/s]"() -> (w141:T4)
              n47 = local write "Moving"(TRUE ("Moving")) -> ()
              n48 = Unbundle By Name(w140) -> ("Go to X"=w127:dbl, "Go to Y"=w128:dbl, "Go to Z"=w131:dbl)
              n49 = Add(x=w131, y=w130) -> (x+y=w129:dbl)
              n50 = Bundle("Go to X"=w127, "Go to Y"=w128, w129) -> (w126:cluster{"Go to X":dbl, "Go to Y":dbl, dbl})  [unwired: 1 in]
              n51 = call "Go2XYZ (SubVI).vi"(".NET Refnum in"=w144, "Go to Coordinates"=w126, "Axis Speeds"=w141, "error in (no error)"=w143) -> (".NET Refnum out"=w139:refnum<k24>, "Final Position"=w137:T11, "error out"=w138:errorcluster)  [unwired: 8 in, 1 out]
              n52 = local write "XYZ Stage Current Position"(w137) -> ()
              n53 = call "Disconnect.vi"("error in (no error)"=w138, "controller"=w139) -> ("error out"=w132:errorcluster)  [unwired: 9 in]
              "Z step" <- w130
            }
            frame #1 {
              n54 = local write "Moving"(FALSE ("Moving")) -> ()
              n55 = Wait (ms)(milliseconds to wait=u32 1000) -> ()  [unwired: 1 out]
            }
            frame #2 {
              # "Collect and analyze image"
              n56 = call <vilib>:"IMAQdx Grab.vi"("error in"=w166, "Image In"=w168, "Session In"=w167) -> ("error out"=w165:errorcluster, "Image Out"=w164:T1)  [unwired: 1 in, 6 out]
              n57 = call "IMAQ Rotate"("error in (no error)"=w165, "Angle (degrees)"=sgl 180.0, "Image Src"=w164) -> ("error out"=w162:errorcluster, "Image Dst Out"=w157:T1)  [unwired: 7 in]
              n58 = local read "Match parameters"() -> (w155:T3)
              n59 = call "IMAQ Histograph"("error in (no error)"=w162, "Image"=w157) -> ("error out"=w161:errorcluster, "Standard  Deviation"=w153:sgl, "Mean Value"=w154:sgl, "Histogram Graph"=→"Intensity histogram":T6)  [unwired: 6 in]
              n60 = local write "Image"(w157) -> ()
              n61 = call "IMAQ LineProfile"("error in (no error)"=w161, "Line Coordinates"="Line Profile Coordinates", "Image"=w157) -> ("error out"=w158:errorcluster, "Line Graph"=→"Line Profile":cluster{"x0":sgl, "dx":sgl, "Pixels Line":sgl[]})  [unwired: 2 in, 2 out]
              n62 = call "IMAQ Match Pattern 4"("Image"=w157, "Template Image"=w156, "Parameters"=w155, "error in (no error)"=w158) -> ("Matches (pixel)"=w152:T2, "Number of Matches"=w151:i32)  [unwired: 7 in, 3 out]
              "Matches (pixel)" <- w152
              n63 = call "AnalyzePatternMatches (SubVI).vi"("Number of Matches"=w151, "Matches (pixel)"=w152) -> ()  [unwired: 6 in, 4 out]
              n64 = local read "Image"() -> ()  [unwired: 1 in]
              n65 = local read "Z step"() -> (w170:dbl)
            }
          }
          n66 = local read "Initial Location [mm]"() -> (w115:T5)
          n67 = Unbundle By Name() -> ()  [unwired: 1 in, 1 out]
          n68 = Unbundle By Name(w115) -> ("Go to Z"=w113:dbl)
          n69 = Add(x=w113, y=w103) -> (x+y=w114:dbl)
        }
        "Z displacement [mm]" <- w91
        n70 = Bundle() -> ()  [unwired: 3 in, 1 out]
        n71 = Bundle() -> ()  [unwired: 3 in, 1 out]
        n72 = Bundle() -> ()  [unwired: 3 in, 1 out]
        n73 = Bundle(w91, w93) -> (→"Mean intensity":cluster{dbl[], sgl[]})  [unwired: 1 in]
        n74 = Bundle(w91, w90) -> (→"SD Intensity":cluster{dbl[], sgl[]})  [unwired: 1 in]
      }
      frame #3 {
        w182 = "_"
        # "Save the results to a file for that XY position setting"
        n75 = local read "Z displacement [mm]"() -> (w187:dbl[])
        n76 = local read "Initial Location [mm]"() -> (w176:T5)
        n77 = Array Size(array=w187) -> (size(s)=w188:i32)
        n78 = for {
          N: w188 -> [_]
          tunnel: [w199] -> w192 mode=indexing
          i -> [w195]
          n79 = local read "True match index vector"() -> (w196:i32[])
          n80 = local read "Z displacement [mm]"() -> (w201:dbl[])
          n81 = local read item#-1() -> ()  [unwired: 1 out]
          n82 = local read item#-1() -> ()  [unwired: 1 out]
          n83 = local read item#-1() -> ()  [unwired: 1 out]
          n84 = local read item#-1() -> (w198)
          n85 = Index Array(array=w201, index=w195) -> (element=w200:dbl)
          n86 = Index Array(array=w198, index=w195) -> (element=w197)
          n87 = Index Array(index=w195) -> ()  [unwired: 1 in, 1 out]
          n88 = Index Array(index=w195) -> ()  [unwired: 1 in, 1 out]
          n89 = Index Array(index=w195) -> ()  [unwired: 1 in, 1 out]
          n90 = Index Array(array=w196, index=w195) -> (element=w194:i32)
          n91 = Build Array(w200, w197, w194) -> (w199:dbl[])  [unwired: 3 in]
        }
        n92 = Unbundle By Name(w176) -> ("Go to X"=w177:dbl, "Go to Y"=w178:dbl, "Go to Z"=w179:dbl)
        n93 = Number To Decimal String(number=w177) -> (decimal integer string=w181:string)  [unwired: 1 in]
        n94 = Number To Decimal String(number=w178) -> (decimal integer string=w183:string)  [unwired: 1 in]
        n95 = Number To Decimal String(number=w179) -> (decimal integer string=w184:string)  [unwired: 1 in]
        n96 = Concatenate Strings("Results_", w181, w182, w183, w182, w184, ".csv" ("string")) -> (w186:string)
        n97 = Build Path(base path="Save plots file path", name or relative path=w186) -> (appended path=w173:path)
        n98 = local read "File delimiter"() -> (w193:string)
        n99 = call-poly <vilib>:"Write Delimited Spreadsheet.vi"("file path (dialog if empty)"=w173, "1D data"=string[] ["Z displacement [mm]", "SD of line profile", "Image mean intensity", "Image SD of intensity", "True match score", "True match index"], "append to file? (new file:F)"=FALSE, "error in (no error)"=w172, "delimiter (\\t)"=w193) -> ("error out"=w191:errorcluster)  [unwired: 9 in, 1 out]
        n100 = call-poly <vilib>:"Write Delimited Spreadsheet.vi"("file path (dialog if empty)"=w173, "2D data"=w192, "append to file? (new file:F)"=TRUE, "error in (no error)"=w191, "delimiter (\\t)"=w193) -> ("error out"=w171:errorcluster)  [unwired: 9 in, 1 out]
      }
    }
    n101 = call <vilib>:"IMAQdx Close Camera.vi"() -> ("error out"=w20:errorcluster)  [unwired: 2 in, 9 out]
    n102 = call "Imaq Dispose"("error in (no error)"=w20) -> ("error out"=w24:errorcluster)  [unwired: 5 in]
    "Coord. Index" <- w22
  }
  n103 = disable-structure shown="Disabled" {
    frame Disabled {
      n104 = call "Vision Assistant"() -> ()  [unwired: 25 in, 3 out]
    }
    frame Enabled {
    }
  }
  n105 = Merge Errors(w6, w1) -> (w5:errorcluster)
  n106 = call <vilib>:"General Error Handler.vi"("error in (no error)"=w5) -> ("error out"=→"Error report":errorcluster)  [unwired: 2 in, 12 out]
